vi "Get Euler Angles.vi"(10 "Received Array":u8[](array[numeric]) format="%02x") -> (1 "Yaw (deg)":dbl, 2 "Pitch (deg)":dbl, 3 "Roll (deg)":dbl)   [LabVIEW 2012]
uses:
  <vilib>/Analysis/NI_AngleConversion.lvlib
panel:
  in  "Command":string="7565 0102 0202 E1C7"
  out "result string":string
  # "7565800E0E0C3DFEFAD33E5CA4DA4031CF5E4033"
  # "75 65 80 0E 0E 0C 3C 3F 71 67 3D 38 04 4E C0 40 45 63 44 6A"
  # "7565 80 0E 0E 0C      3C3F7167    3D38044E     C0404563      446A\n7565800E0E0C3C3F655F3D381B48C04045E2C095\n7565800E0E0C3C3EB4673D37C64AC04045F1D1FC\n7565800E0E0C3C3EEC5A3D37C14AC04046070EB1\n7565800E0E0C3C3F2ACB3D378B53C040450F9810"
  # "YAW C0404563"
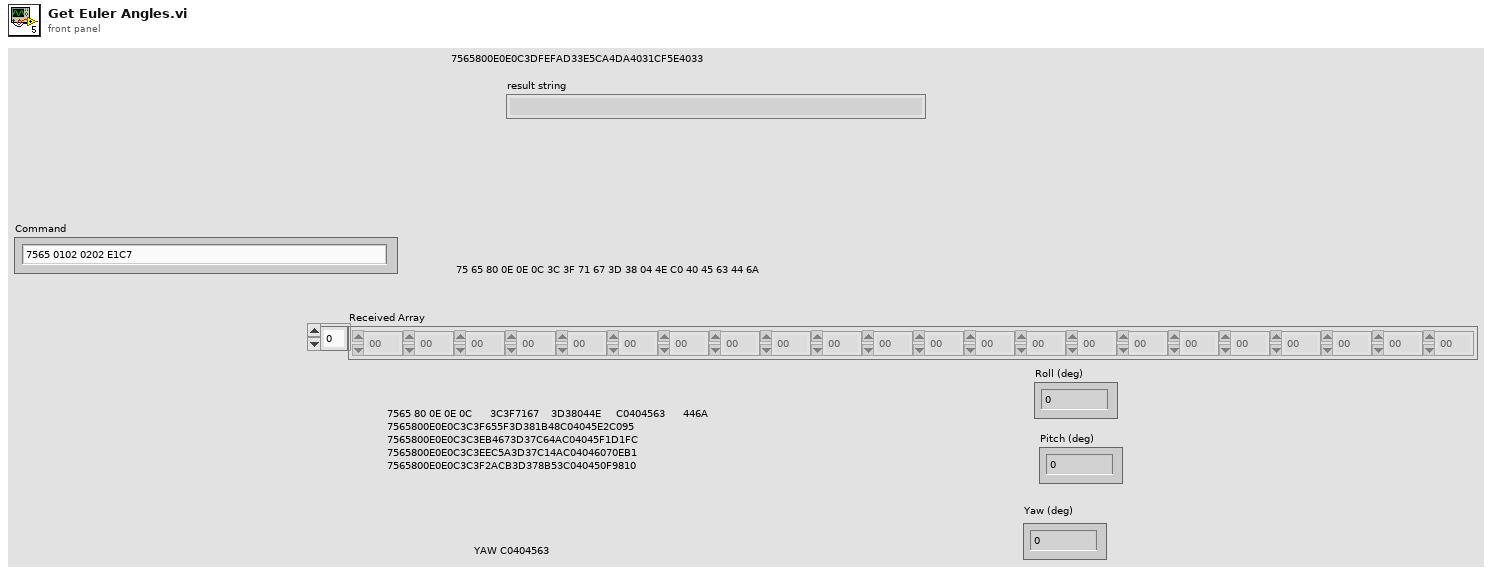
[diagram p1: front panel]
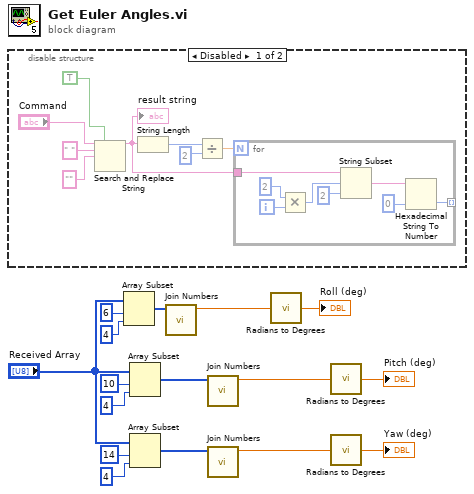
[diagram p0: block diagram]
diagram:
  n1 = disable-structure shown="Disabled" {
    frame Disabled {
      n2 = Search and Replace String(replace all?=TRUE ("replace all? (F)"), input string="Command", search string=" ", replace string="" ("replace string (\"\")")) -> (result string=w20:string)  [unwired: 4 in, 3 out]
      "result string" <- w20
      n3 = String Length(string=w20) -> (length=w19:i32)
      n4 = Divide(x=w19, y=2) -> (x/y=w17:dbl)
      n5 = for {
        N: w17 -> [_]
        tunnel: w20 -> [w32]
        tunnel: [w25] -> _ mode=indexing
        i -> [w30]
        n6 = Multiply(x=2, y=w30) -> (x*y=w28:i32)
        n7 = String Subset(string=w32, offset (0)=w28, length (rest)=2 ("length (rest)")) -> (substring=w27:string)
        n8 = Hexadecimal String To Number(string=w27, default (0uL)=u8 0 ("default (0 U32)")) -> (number=w25:u8)  [unwired: 1 in, 1 out]
      }
    }
    frame Enabled {
    }
  }
  n9 = Array Subset(array="Received Array", index=6, length=4) -> (w8:u8[])
  n10 = Array Subset(array="Received Array", index=10, length=4) -> (w10:u8[])
  n11 = Array Subset(array="Received Array", index=14, length=4) -> (w9:u8[])
  n12 = call "Join Numbers.vi"("Array of 4 U8"=w8) -> ("Single-Precision Float"=w6:sgl)  [unwired: 10 in]
  n13 = call "Join Numbers.vi"("Array of 4 U8"=w10) -> ("Single-Precision Float"=w1:sgl)  [unwired: 10 in]
  n14 = call "Join Numbers.vi"("Array of 4 U8"=w9) -> ("Single-Precision Float"=w4:sgl)  [unwired: 10 in]
  n15 = call <vilib>:"Radians to Degrees.vi"("Radians"=w6) -> ("Degrees"=→"Roll (deg)":dbl)
  n16 = call <vilib>:"Radians to Degrees.vi"("Radians"=w1) -> ("Degrees"=→"Pitch (deg)":dbl)
  n17 = call <vilib>:"Radians to Degrees.vi"("Radians"=w4) -> ("Degrees"=→"Yaw (deg)":dbl)
